vi "BP FilterI16_Fast.vi"(3 "Filter":T1, 6 "Array in":i16[][](array[numeric])) -> (0 "Filtered X":dbl[][](array[numeric]))   [LabVIEW 2022 SP3]
uses:
  <vilib>/Analysis/2dsp.llb/1D Convolution (DBL).vi
  <vilib>/Analysis/NI_AALPro.lvlib
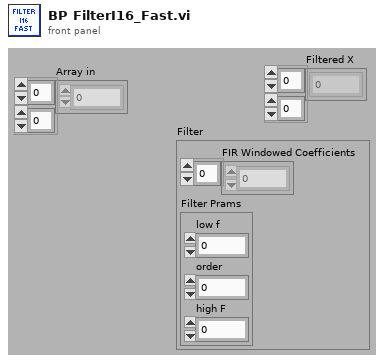
[diagram p1: front panel]
types:
  T1 = cluster{"FIR Windowed Coefficients":dbl[], "Filter Prams":cluster{"low f":i32, "order":i32, "high F":i32}}
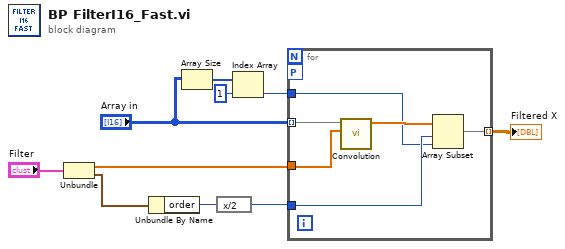
[diagram p0: block diagram]
diagram:
  n1 = Unbundle("Filter") -> ("FIR Windowed Coefficients"=w1:dbl[], "Filter Prams"=w2:cluster{"low f":i32, "order":i32, "high F":i32})
  n2 = Unbundle By Name(w2) -> ("order"=w9:i32)
  n3 = Array Size(array="Array in") -> (size(s)=w6:i32[])
  n4 = expression code="x/2"(w9) -> (w8:i32)
  n5 = Index Array(array=w6, index=1) -> (element=w4:i32)
  n6 = for {
    tunnel: w8 -> [w12]
    tunnel: [w16] -> w10 mode=indexing
    tunnel: "Array in" -> [w15] mode=indexing
    workers-P: _ -> [_]
    tunnel: w1 -> [w14]
    tunnel: w4 -> [w11]
    n7 = call-poly <vilib>:"Convolution.vi"("Y"=w14, "X"=w15) -> ("X * Y"=w13:dbl[])  [unwired: 1 in, 8 out]
    n8 = Array Subset(array=w13, index=w12, length=w11) -> (w16:dbl[])
  }
  "Filtered X" <- w10
